vi "Rank Candidates.vi"(0 "Focus and Tracking":T5, 5 "System of Reference Interface":T6, 7 "Tip":T4, 9 "Calibration":T3, 11 "error in (no error)":errorcluster, 12 "Distance Coeff":dbl=0.5, 13 "Area Coeff":dbl=0.25, 14 "Contrast Coeff":dbl=0.25) -> (4 "Coords [um]":T2(array[cluster]), 6 "Scores":dbl[](array[numeric]), 8 "Visible Objects [pix]":T1(array[cluster]), 15 "error out":errorcluster)   [LabVIEW 2012, in "Targeting Unit.lvlib"]
uses:
  Targeting Unit.lvlib
  <vilib>/Analysis/Matrix/Datatypes/RealMatrix.ctl
  <vilib>/Analysis/Matrix/NI_Matrix.lvlib
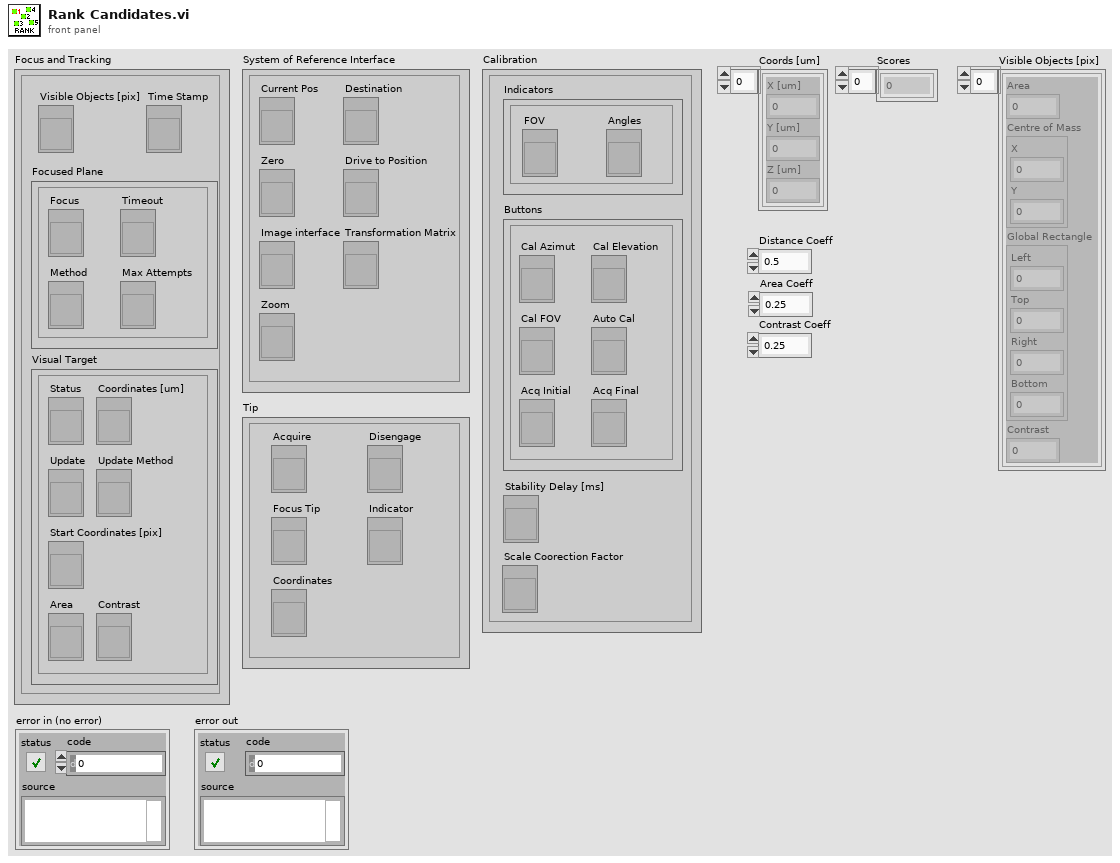
[diagram p1: front panel]
types:
  T1 = cluster{"Area":dbl, "Centre of Mass":cluster{"X":dbl, "Y":dbl}, "Global Rectangle":cluster{"Left":dbl, "Top":dbl, "Right":dbl, "Bottom":dbl}, "Contrast":dbl}[]
  T2 = cluster{"X [um]":dbl, "Y [um]":dbl, "Z [um]":dbl}[]
  T3 = cluster{"Indicators":cluster{"FOV":refnum<vi>, "Angles":refnum<vi>}, "Buttons":cluster{"Cal FOV":refnum<vi>, "Cal Azimut":refnum<vi>, "Cal Elevation":refnum<vi>, "Auto Cal":refnum<vi>, "Acq Initial":refnum<vi>, "Acq Final":refnum<vi>}, "Stability Delay [ms]":refnum<vi>, "Scale Coorection Factor":refnum<vi>}
  T4 = cluster{"Coordinates":refnum<vi>, "Acquire":refnum<vi>, "Disengage":refnum<vi>, "Indicator":refnum<vi>, "Focus Tip":refnum<vi>}
  T5 = cluster{"Focused Plane":cluster{"Focus":refnum<vi>, "Timeout":refnum<vi>, "Max Attempts":refnum<vi>, "Method":refnum<vi>}, "Time Stamp":refnum<vi>, "Visual Target":cluster{"Coordinates [um]":refnum<vi>, "Status":refnum<vi>, "Update":refnum<vi>, "Update Method":refnum<vi>, "Start Coordinates [pix]":refnum<vi>, "Area":refnum<vi>, "Contrast":refnum<vi>}, "Visible Objects [pix]":refnum<vi>}
  T6 = cluster{"Current Pos":refnum<vi>, "Image interface":refnum<vi>, "Transformation Matrix":refnum<vi>, "Zero":refnum<vi>, "Destination":refnum<vi>, "Drive to Position":refnum<vi>, "Zoom":refnum<vi>}
  T7 = cluster{"X [um]":dbl, "Y [um]":dbl, "Z [um]":dbl}
  T8 = typedef "NI_Matrix.lvlib/RealMatrix.ctl" = dbl[][]
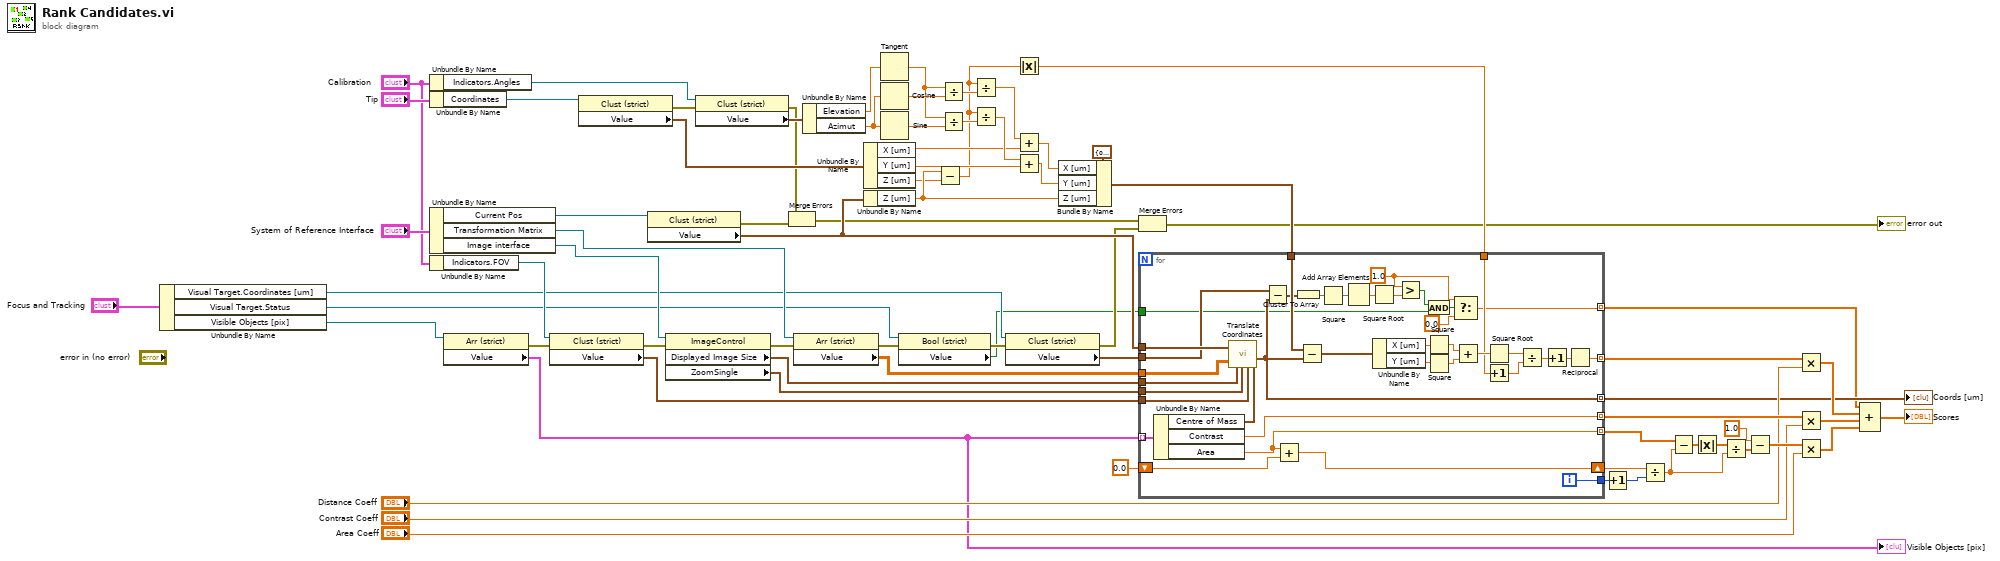
[diagram p0: block diagram]
diagram:
  n1 = Unbundle By Name("Focus and Tracking") -> ("Visual Target.Coordinates [um]"=w6:refnum<vi>, "Visual Target.Status"=w8:refnum<vi>, "Visible Objects [pix]"=w73:refnum<vi>)
  n2 = Unbundle By Name("Calibration") -> ("Indicators.Angles"=w67:refnum<vi>)
  n3 = Unbundle By Name("Tip") -> ("Coordinates"=w71:refnum<vi>)
  n4 = Unbundle By Name("System of Reference Interface") -> ("Current Pos"=w13:refnum<vi>, "Transformation Matrix"=w12:refnum<vi>, "Image interface"=w11:refnum<vi>)
  n5 = Unbundle By Name("Calibration") -> ("Indicators.FOV"=w50:refnum<vi>)
  n6 = property class="Arr (strict)"(reference=w73) -> (error out=w44:errorcluster, "Value"=w19:T1)  [unwired: 1 in, 1 out]
  "Visible Objects [pix]" <- w19
  n7 = property class="Clust (strict)"(reference=w50, error in=w44) -> (error out=w45:errorcluster, "Value"=w70:cluster{"FOVx [um]":dbl, "FOVy [um]":dbl})  [unwired: 1 out]
  n8 = property class="Clust (strict)"(reference=w71) -> (error out=w47:errorcluster, "Value"=w58:T7)  [unwired: 1 in, 1 out]
  n9 = property class="Clust (strict)"(reference=w13) -> (error out=w32:errorcluster, "Value"=w46:T7)  [unwired: 1 in, 1 out]
  n10 = property class="ImageControl"(reference=w11, error in=w45) -> (error out=w68:errorcluster, "Displayed Image Size"=w14:cluster{"Width":u32, "Height":u32}, "ZoomSingle"=w15:cluster{"X":sgl, "Y":sgl})  [unwired: 1 out]
  n11 = property class="Clust (strict)"(reference=w67, error in=w47) -> (error out=w31:errorcluster, "Value"=w66:cluster{"Azimut":dbl, "Elevation":dbl})  [unwired: 1 out]
  n12 = Merge Errors(w31, w32) -> (w33:errorcluster)
  n13 = property class="Arr (strict)"(reference=w12, error in=w68) -> (error out=w9:errorcluster, "Value"=w69:T8)  [unwired: 1 out]
  n14 = Unbundle By Name(w66) -> ("Elevation"=w64:dbl, "Azimut"=w65:dbl)
  n15 = Unbundle By Name(w58) -> ("X [um]"=w55:dbl, "Y [um]"=w56:dbl, "Z [um]"=w18:dbl)
  n16 = Unbundle By Name(w46) -> ("Z [um]"=w48:dbl)
  n17 = Tangent(1:w64) -> (0:w62:dbl)
  n18 = Cosine(x=w65) -> (cos(x)=w63:dbl)
  n19 = Sine(x=w65) -> (sin(x)=w61:dbl)
  n20 = property class="Bool (strict)"(reference=w8, error in=w9) -> (error out=w7:errorcluster, "Value"=w3:bool)  [unwired: 1 out]
  n21 = Subtract(x=w48, y=w18) -> (x-y=w17:dbl)
  n22 = Divide(x=w62, y=w63) -> (x/y=w60:dbl)
  n23 = Divide(x=w62, y=w61) -> (x/y=w59:dbl)
  n24 = Divide(x=w17, y=w60) -> (x/y=w54:dbl)
  n25 = Divide(x=w17, y=w59) -> (x/y=w57:dbl)
  n26 = property class="Clust (strict)"(reference=w6, error in=w7) -> (error out=w5:errorcluster, "Value"=w4:cluster{"X":dbl, "Y":dbl, "Z":dbl})  [unwired: 1 out]
  n27 = Absolute Value(x=w17) -> (abs(x)=w16:dbl)
  n28 = Add(x=w54, y=w55) -> (x+y=w53:dbl)
  n29 = Add(x=w57, y=w56) -> (x+y=w52:dbl)
  n30 = Bundle By Name(cluster=T7 {"X [um]"=0.0, "Y [um]"=0.0, "Z [um]"=0.0} ("Target Coordinates"), "X [um]"=w53, "Y [um]"=w52, "Z [um]"=w48) -> (w51:T7)
  n31 = Merge Errors(w33, w5) -> (→"error out":errorcluster)
  n32 = for {
    tunnel: w19 -> [w113] mode=indexing
    tunnel: w70 -> [w93]
    tunnel: w46 -> [w98]
    tunnel: w69 -> [w83]
    tunnel: w51 -> [w112]
    shift-right: [w104] -> w41
    shift-left: 0.0 -> [w103]
    tunnel: [w102] -> w42 mode=indexing
    tunnel: [w101] -> w40
    tunnel: [w100] -> w27 mode=indexing
    tunnel: [w99] -> w29 mode=indexing
    tunnel: [w89] -> w10 mode=indexing
    tunnel: w16 -> [w90]
    tunnel: w15 -> [w96]
    tunnel: w14 -> [w95]
    tunnel: w4 -> [w88]
    tunnel: w3 -> [w77]
    tunnel: [w76] -> w2 mode=indexing
    i -> [w101]
    w79 = 1.0 ("x")
    n33 = Unbundle By Name(w113) -> ("Centre of Mass"=w97:cluster{"X":dbl, "Y":dbl}, "Contrast"=w99:dbl, "Area"=w102:dbl)
    n34 = call "Translate Coordinates.vi"("Transformation Matrix"=w83, "Coordinates [pix]"=w97, "FOV"=w93, "Visualiser Zoom"=w96, "Scope Position"=w98, "Image Area"=w95) -> ("Target Coordinates"=w89:T7)  [unwired: 4 in, 1 out]
    n35 = Subtract(x=w88, y=w89) -> (x-y=w87:cluster{dbl, dbl, dbl})
    n36 = Add(x=w102, y=w103) -> (x+y=w104:dbl)
    n37 = Cluster To Array(cluster=w87) -> (array=w86:dbl[])
    n38 = Subtract(x=w112, y=w89) -> (x-y=w111:T7)
    n39 = Square(x=w86) -> (x^2=w85:dbl[])
    n40 = Add Array Elements(numeric array=w85) -> (sum=w84:dbl)
    n41 = Square Root(x=w84) -> (sqrt(x)=w82:dbl)
    n42 = Unbundle By Name(w111) -> ("X [um]"=w110:dbl, "Y [um]"=w109:dbl)
    n43 = Greater?(x=w79, y=w82) -> (0:w78:bool)
    n44 = And(x=w78, y=w77) -> (x .and. y?=w80:bool)
    n45 = Square(x=w110) -> (x^2=w108:dbl)
    n46 = Square(x=w109) -> (x^2=w107:dbl)
    n47 = Select(t=w79, s=w80, f=0.0) -> (s? t:f=w76:dbl)
    n48 = Add(x=w108, y=w107) -> (x+y=w106:dbl)
    n49 = Square Root(x=w106) -> (sqrt(x)=w94:dbl)
    n50 = Increment(x=w90) -> (x+1=w91:dbl)
    n51 = Divide(x=w94, y=w91) -> (x/y=w92:dbl)
    n52 = Increment(x=w92) -> (x+1=w105:dbl)
    n53 = Reciprocal(x=w105) -> (1/x=w100:dbl)
  }
  "Coords [um]" <- w10
  n54 = Increment(x=w40) -> (x+1=w39:i32)
  n55 = Divide(x=w41, y=w39) -> (x/y=w36:dbl)
  n56 = Subtract(x=w42, y=w36) -> (x-y=w38:dbl[])
  n57 = Absolute Value(x=w38) -> (abs(x)=w37:dbl[])
  n58 = Divide(x=w37, y=w36) -> (x/y=w34:dbl[])
  n59 = Subtract(x=1.0, y=w34) -> (x-y=w28:dbl[])
  n60 = Multiply(x=w27, y="Distance Coeff") -> (x*y=w23:dbl[])
  n61 = Multiply(x=w29, y="Contrast Coeff") -> (x*y=w22:dbl[])
  n62 = Multiply(x=w28, y="Area Coeff") -> (x*y=w21:dbl[])
  n63 = Compound Arithmetic op=ADD(w2, w23, w22, w21) -> (→"Scores":dbl[])
